vi "encodeStream.vi"(8 "error in (no error)":errorcluster, 11 "tBSONRegEx in":refnum<class "tBSONRegEx.lvclass">) -> (0 "error out":errorcluster, 2 "Byte Array":u8[](array[numeric]), 3 "tBSONRegEx out":refnum<class "tBSONRegEx.lvclass">)   [LabVIEW 2013, in "BSON.lvlib" / "tBSONRegEx.lvclass"]
uses:
  tBSONRegEx.lvclass
  tBSONElement/tBSONElement.lvclass
  getRegularExpression.vi
  getOptionsString.vi
  BSON.lvlib
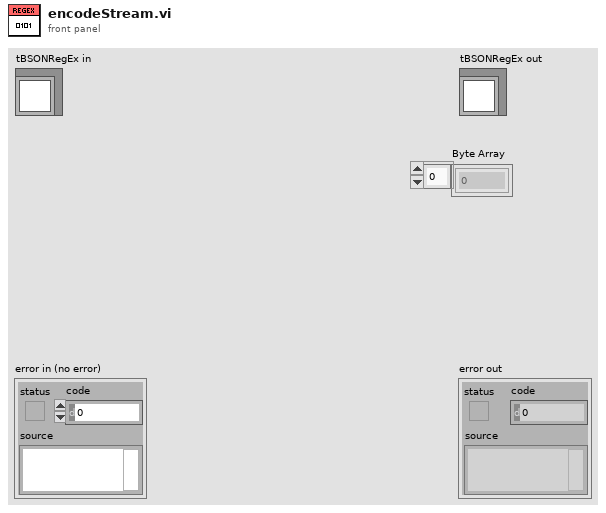
[diagram p1: front panel]
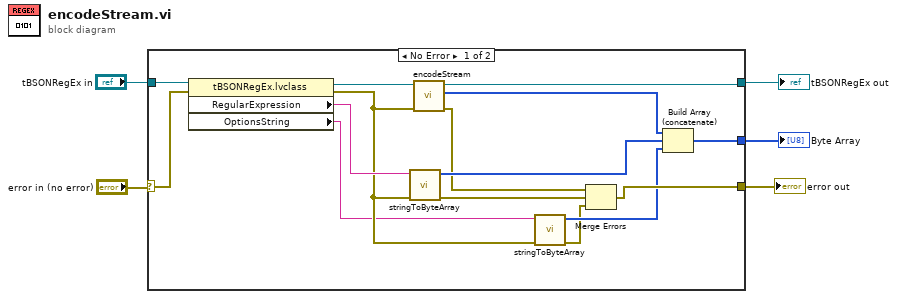
[diagram p0: block diagram]
diagram:
  n1 = case shown="No Error" "error in (no error)" {
    selector: "error in (no error)" -> [w19 w21]
    tunnel: "tBSONRegEx in" -> [w20 w22]
    tunnel: [w7 w22] -> w1
    tunnel: [w17 w21] -> w2
    tunnel: [w18 _] -> w5
    frame No Error {
      n2 = property class="tBSONRegEx.lvclass"(reference=w20, error in=w19) -> (reference out=w11:refnum<class "tBSONRegEx.lvclass">, error out=w10:errorcluster, "RegularExpression"=w16:string, "OptionsString"=w6:string)
      n3 = call "stringToByteArray.vi"("error in (no error)"=w10, "String"=w16) -> ("error out"=w15:errorcluster, "byte array"=w14:u8[])  [unwired: 8 in]
      n4 = call-parent "encodeStream.vi"("error in (no error)"=w10, "tBSONElement in"=w11) -> ("error out"=w8:errorcluster, "Byte Array"=w9:u8[], "tBSONElement out"=w7:refnum<class "tBSONRegEx.lvclass">)  [unwired: 7 in]
      n5 = call "stringToByteArray.vi"("error in (no error)"=w10, "String"=w6) -> ("error out"=w12:errorcluster, "byte array"=w13:u8[])  [unwired: 8 in]
      n6 = Merge Errors(w8, w15, w12) -> (w17:errorcluster)
      n7 = Build Array (concatenate)(w9, w14, w13) -> (w18:u8[])
    }
    frame Error {
    }
  }
  "error out" <- w2
  "tBSONRegEx out" <- w1
  "Byte Array" <- w5
